vi "Setup and move.vi"(7 "Motor params":T1={"Motor type"=enum."Unipolar", "Direction"=enum."CW", "Steps"=1000, "Frequency (Hz)"=127, "Step type"=enum."Full"}, 8 "error in (no error)":errorcluster, 9 "Ángulo":dbl format="%#_g°", 10 "Direction":T2=enum."CW", 11 "Arduino Mod ID":i32) -> (0 "error out":errorcluster)   [LabVIEW 2020]
uses:
  Arduino_stepper/Libraries/Arduino stepper/Arduino stepper.lvlib
  Arduino_stepper/Libraries/Arduino stepper/Support/Motor direction -- enum.ctl
  Arduino_stepper/Libraries/Arduino stepper/Support/Motor parameters.ctl
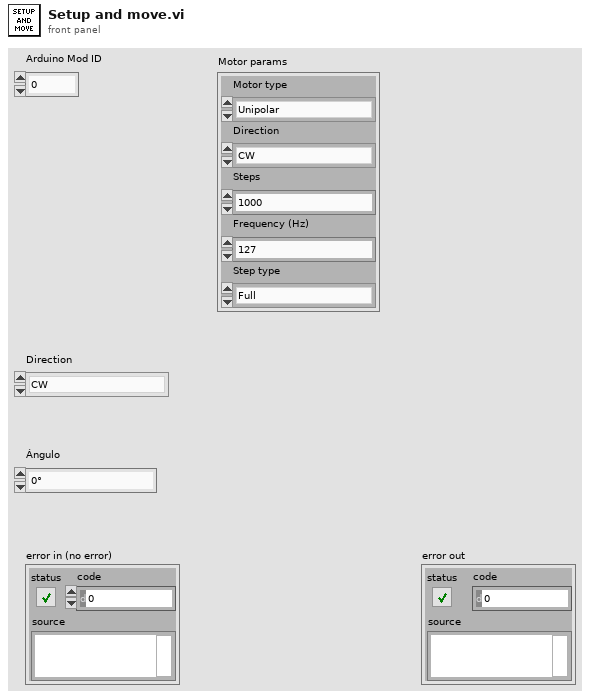
[diagram p1: front panel]
types:
  T1 = typedef "Arduino stepper.lvlib/Motor parameters.ctl" = cluster{"Motor type":enum8{"", "Unipolar", "Bipolar"}, "Direction":T2, "Steps":u16, "Frequency (Hz)":u8, "Step type":enum8{"", "Half", "Full"}}
  T2 = typedef "Arduino stepper.lvlib/Motor direction -- enum.ctl" = enum8{"", "CW", "CCW"}
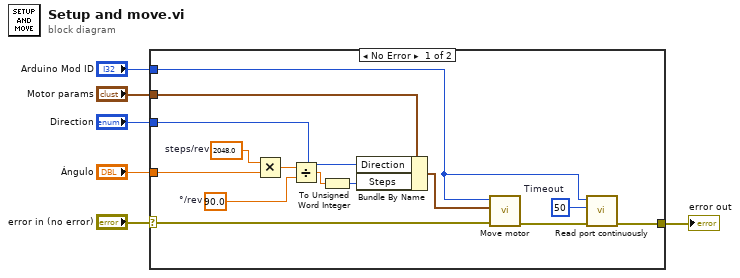
[diagram p0: block diagram]
diagram:
  n1 = case shown="No Error" "error in (no error)" {
    selector: "error in (no error)" -> [w8 w21]
    tunnel: "Direction" -> [w20 _]
    tunnel: "Arduino Mod ID" -> [w19 _]
    tunnel: [w17 w21] -> w5
    tunnel: "Ángulo" -> [w9 _]
    tunnel: "Motor params" -> [w7 _]
    frame No Error {
      w18 = 50  # Timeout
      w12 = 90.0  # °/rev
      w10 = 2048.0  # steps/rev
      n2 = Multiply(x=w10, y=w9) -> (x*y=w11:dbl)
      n3 = Divide(x=w11, y=w12) -> (x/y=w13:dbl)
      n4 = To Unsigned Word Integer(number=w13) -> (unsigned 16bit integer=w14:u16)
      n5 = Bundle By Name(cluster=w7, "Direction"=w20, "Steps"=w14) -> (w15:T1)
      n6 = call "Move motor.vi"("error in"=w8, "Motor params"=w15, "Module ID"=w19) -> ("error out"=w16:errorcluster)  [unwired: 8 in]
      n7 = call "Read port continuously.vi"("error in"=w16, "Timeout"=w18, "Module ID"=w19) -> ("error out"=w17:errorcluster)  [unwired: 8 in]
    }
    frame Error {
    }
  }
  "error out" <- w5
